vi "pressure control.vi"() -> ()   [LabVIEW 2019]
panel:
  in  "Slide":dbl(slide) scale=0.0..5.0
  out "Voltage":dbl format="%.4f"
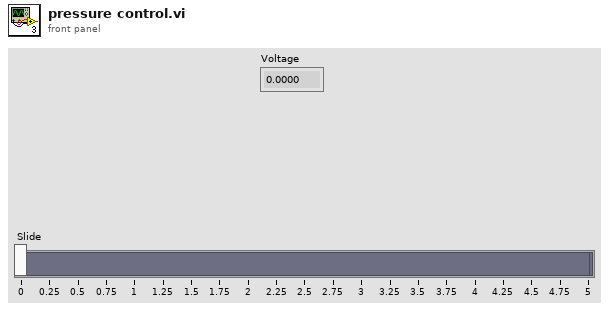
[diagram p1: front panel]
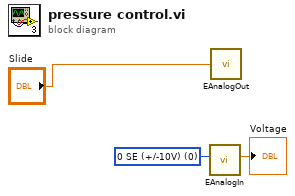
[diagram p0: block diagram]
diagram:
  w2 = u16 0 items=["0 SE (+/-10V)", "1 SE (+/-10V)", "2 SE (+/-10V)", "3 SE (+/-10V)", "4 SE (+/-10V)", "5 SE (+/-10V)", "6 SE (+/-10V)", "7 SE (+/-10V)", "0-1 Diff", "2-3 Diff", "4-5 Diff", "6-7 Diff"] ("Channel")
  n1 = call <vilib>:"EAnalogIn.vi"("Channel"=w2) -> ("Voltage"=→"Voltage":dbl)  [unwired: 6 in, 4 out]
  n2 = call <vilib>:"EAnalogOut.vi"("Analog Output 0 [volts]"="Slide") -> ()  [unwired: 13 in, 2 out]
